vi "Verify Member Data Against Database.vi"(8 "error in (no error)":errorcluster, 11 "Field in":refnum<class "Field.lvclass">) -> (0 "error out":errorcluster, 3 "Field out":refnum<class "Field.lvclass">)   [LabVIEW 2020, in "Old Field.lvlib" / "Field.lvclass"]
uses:
  Field.lvclass
  Field.lvclass/Field.ctl
  Database Libraries/Database/Database Class/Database.lvclass
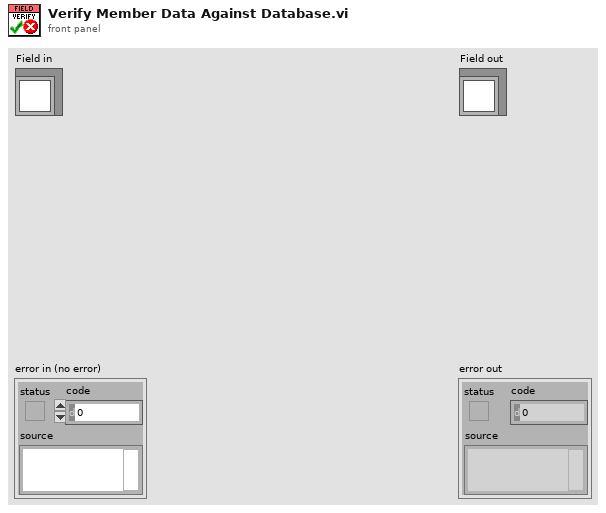
[diagram p1: front panel]
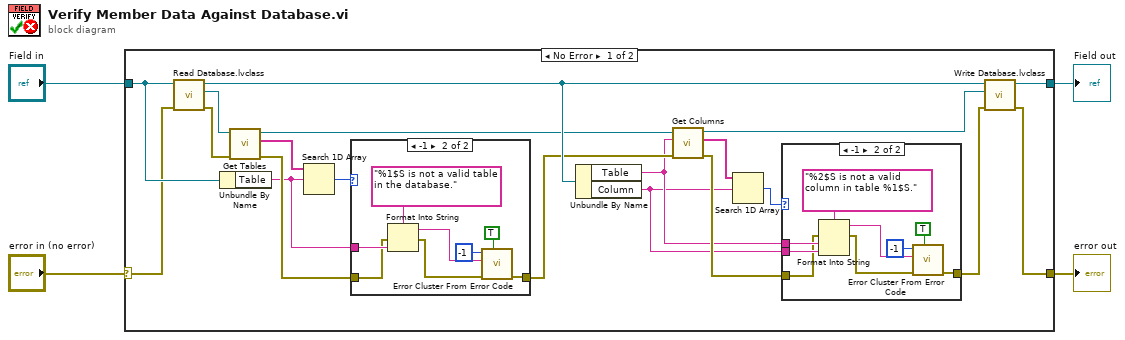
[diagram p0: block diagram]
diagram:
  n1 = case shown="No Error" "error in (no error)" {
    selector: "error in (no error)" -> [w5 w45]
    tunnel: [w8 w45] -> w3
    tunnel: [w20 w44] -> w1
    tunnel: "Field in" -> [w18 w44]
    frame No Error {
      n2 = call "Read Database.lvclass.vi"("error in (no error)"=w5, "Field in"=w18) -> ("error out"=w23:errorcluster, "Database.lvclass"=w24:refnum<class "Database.lvclass">, "Field out"=w14:refnum<class "Field.lvclass">)  [unwired: 7 in]
      n3 = Unbundle By Name(w18) -> ("Table"=w17:string)
      n4 = call-dynamic "Get Tables.vi"("error in (no error)"=w23, "Database in"=w24) -> ("error out"=w19:errorcluster, "Table Names"=w22:string[], "Database out"=w13:refnum<class "Database.lvclass">)  [unwired: 7 in]
      n5 = Search 1D Array(1D array=w22, element=w17) -> (index of element=w21:i32)  [unwired: 1 in]
      n6 = case shown="-1" w21 {
        tunnel: w19 -> [w35 w41]
        tunnel: [w35 w38] -> w12
        tunnel: w17 -> [_ w42]
        frame 0, Default {
        }
        frame -1 {
          n7 = Format Into String(format string="%1$S is not a valid table in the database.", error in=w41, w42) -> (resulting string=w39:string, error out=w40:errorcluster)  [unwired: 1 in]
          n8 = call <vilib>:"Error Cluster From Error Code.vi"("show call chain? (False)"=TRUE, "error in (no error)"=w40, "error message (\"\")"=w39, "error code (0)"=-1) -> ("error out"=w38:errorcluster)  [unwired: 5 in]
        }
      }
      n9 = Unbundle By Name(w14) -> ("Table"=w7:string, "Column"=w6:string)
      n10 = call-dynamic "Get Columns.vi"("error in (no error)"=w12, "Table Name"=w7, "Database in"=w13) -> ("error out"=w11:errorcluster, "Column Name Array"=w15:string[], "Database out"=w10:refnum<class "Database.lvclass">)  [unwired: 6 in]
      n11 = Search 1D Array(1D array=w15, element=w6) -> (index of element=w16:i32)  [unwired: 1 in]
      n12 = case shown="-1" w16 {
        tunnel: [w25 w31] -> w9
        tunnel: w7 -> [_ w28]
        tunnel: w11 -> [w25 w26]
        tunnel: w6 -> [_ w27]
        frame 0, Default {
        }
        frame -1 {
          n13 = Format Into String(format string="%2$S is not a valid column in table %1$S.", error in=w26, w28, w27) -> (resulting string=w32:string, error out=w33:errorcluster)  [unwired: 1 in]
          n14 = call <vilib>:"Error Cluster From Error Code.vi"("show call chain? (False)"=TRUE, "error in (no error)"=w33, "error message (\"\")"=w32, "error code (0)"=-1) -> ("error out"=w31:errorcluster)  [unwired: 5 in]
        }
      }
      n15 = call "Write Database.lvclass.vi"("error in (no error)"=w9, "Database.lvclass"=w10, "Field in"=w14) -> ("error out"=w8:errorcluster, "Field out"=w20:refnum<class "Field.lvclass">)  [unwired: 7 in]
    }
    frame Error {
    }
  }
  "error out" <- w3
  "Field out" <- w1
